vi "Get Min Meter Value.vi"(8 "error in (no error)":errorcluster, 11 "Item Ref in":T1 format="%.0x") -> (0 "error out":errorcluster, 2 "Min Gauge Value":dbl, 3 "Item Ref out":T1 format="%.0x")   [LabVIEW 2011, in "Meter Detection Custom Device.lvlib"]
uses:
  Meter Detection Custom Device.lvlib
  <vilib>/NI Veristand/Custom Device API/Custom Device Item Ref.ctl
  Meter Detection Global Variable.vi
  <vilib>/NI Veristand/Custom Device API/Get Item Property (Double).vi
  <vilib>/NI Veristand/Custom Device API/Custom Device API.lvlib
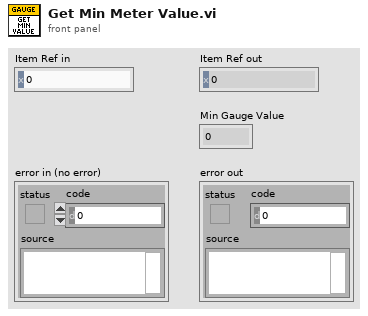
[diagram p1: front panel]
types:
  T1 = typedef "Custom Device API.lvlib/Custom Device Item Ref.ctl" = u64
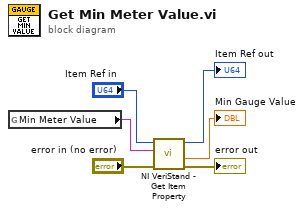
[diagram p0: block diagram]
diagram:
  n1 = global read "Meter Detection Global Variable.vi" "Min Meter Value"() -> (w1:string)
  n2 = call-poly <vilib>:"NI VeriStand - Get Item Property.vi"("error in (no error)"="error in (no error)", "Property Name"=w1, "Item Ref in"="Item Ref in") -> ("error out"=→"error out":errorcluster, "Value"=→"Min Gauge Value":dbl, "Item Ref out"=→"Item Ref out":T1)  [unwired: 5 in, 1 out]
